vi "Teleop - CP Up Down (SubVI).vi"(11 "Raise / Lower Cylinder":bool) -> (3 "controlPanelCylinder":enum16{"off", "on", "forward", "back"}(ring))   [LabVIEW 2019]
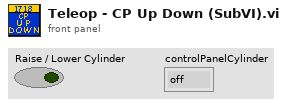
[diagram p1: front panel]
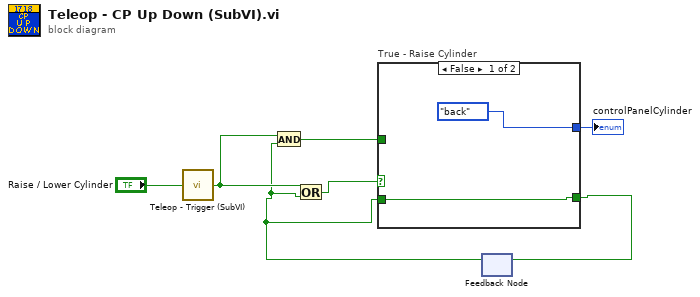
[diagram p0: block diagram]
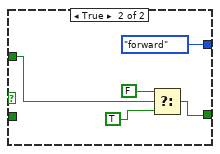
[diagram p2: hidden frame]
diagram:
  n1 = call "Teleop - Trigger (SubVI).vi"("Trigger"="Raise / Lower Cylinder") -> ("Trigger Output"=w3:bool)
  n2 = feedback #1() -> (w1:bool)  [unwired: 1 in]
  n3 = And(x=w3, y=w1) -> (x .and. y?=w2:bool)
  n4 = Or(x=w3, y=w1) -> (x .or. y?=w5:bool)
  n5 = case "True - Raise Cylinder" shown="False" w5 {
    tunnel: [enum16{"off", "on", "forward", "back"}."back" ("controlPanelCylinder") enum16{"off", "on", "forward", "back"}."forward" ("controlPanelCylinder")] -> w6
    tunnel: [w8 w13] -> w4
    tunnel: w2 -> [_ w12]
    tunnel: w1 -> [w8 _]
    frame False {
    }
    frame True {
      n6 = Select(t=FALSE, s=w12, f=TRUE ("Raise / Lower Cylinder")) -> (s? t:f=w13:bool)
    }
  }
  "controlPanelCylinder" <- w6
  n7 = feedback-in #1(w4) -> ()
